vi "cache tag indices.vi"(8 "error in":errorcluster, 9 "index cluster":variant, 10 "channel classification":T1, 11 "Temperature Controller Logic runtime in":refnum<class "Temperature Controller Logic runtime.lvclass">) -> (0 "error out":errorcluster, 3 "Temperature Controller Logic runtime out":refnum<class "Temperature Controller Logic runtime.lvclass">)   [LabVIEW 2013, in "Temperature Controller Logic runtime.lvclass"]
uses:
  Temperature Controller Logic runtime.lvclass
  <vilib>/NI/Tag Bus Module Framework/channel/channel classification.ctl
  configuration/parameter data indices.ctl
  Temperature Controller Logic runtime.lvclass/Temperature Controller Logic runtime.ctl
  configuration/result data indices.ctl
  configuration/Temperature Controller Logic configuration.lvclass
  <vilib>/NI/Tag Bus Module Framework/channel/TBM channel.lvclass
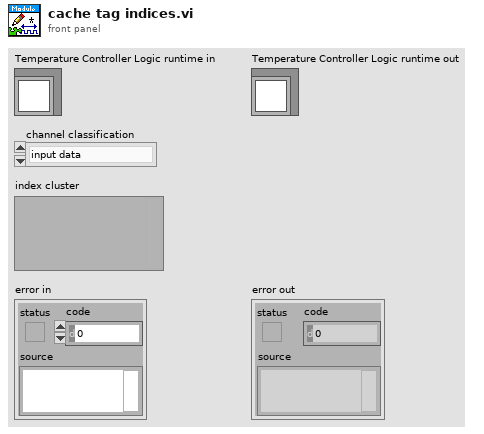
[diagram p1: front panel]
types:
  T1 = typedef "TBM channel.lvclass/channel classification.ctl" = enum16{"input data", "output data", "processing parameter", "processing result"}
  T2 = typedef "Temperature Controller Logic configuration.lvclass/parameter data indices.ctl" = cluster{"Double.Temperature":i32, "Double.setpoint":i32, "Double.output range high":i32, "Double.output range low":i32, "Double.Kc":i32, "Double.Ti":i32, "Double.Td":i32, "Boolean.Fan on?":i32}
  T3 = typedef "Temperature Controller Logic configuration.lvclass/result data indices.ctl" = cluster{"Double.fan":i32, "Double.lamp":i32}
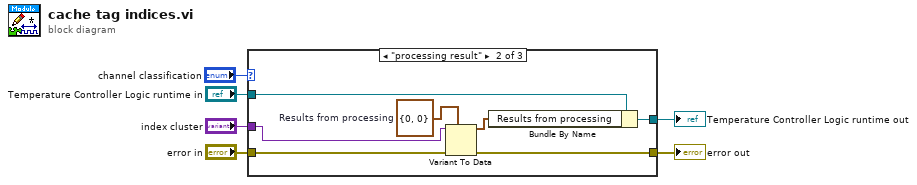
[diagram p0: block diagram]
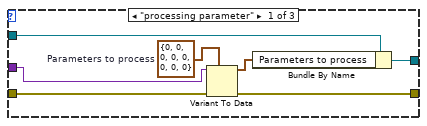
[diagram p2: hidden frame]
diagram:
  n1 = case shown="\"processing result\"" "channel classification" {
    tunnel: "index cluster" -> [w12 w19 _]
    tunnel: [w11 w18 w22] -> w2
    tunnel: "Temperature Controller Logic runtime in" -> [w10 w17 w22]
    tunnel: "error in" -> [w9 w16 w21]
    tunnel: [w8 w15 w21] -> w1
    frame "processing parameter" {
      w7 = T2 {"Double.Temperature"=0, "Double.setpoint"=0, "Double.output range high"=0, "Double.output range low"=0, "Double.Kc"=0, "Double.Ti"=0, "Double.Td"=0, "Boolean.Fan on?"=0}  # Parameters to process
      n2 = Variant To Data(error in=w9, type=w7, Variant=w12) -> (data=w13:T2, error out=w8:errorcluster)
      n3 = Bundle By Name(cluster=w10, "Parameters to process"=w13) -> (w11:refnum<class "Temperature Controller Logic runtime.lvclass">)
    }
    frame "processing result" {
      w14 = T3 {"Double.fan"=0, "Double.lamp"=0}  # Results from processing
      n4 = Variant To Data(error in=w16, type=w14, Variant=w19) -> (data=w20:T3, error out=w15:errorcluster)
      n5 = Bundle By Name(cluster=w17, "Results from processing"=w20) -> (w18:refnum<class "Temperature Controller Logic runtime.lvclass">)
    }
    frame Default {
    }
  }
  "error out" <- w1
  "Temperature Controller Logic runtime out" <- w2
